vi "UDP_choosen_string_to_DBL.vi"(4 "main ID":i32, 5 "secondary ID":i32, 6 "Data to read":T1, 7 "input string":string) -> (3 "output number":dbl)   [LabVIEW 2012]
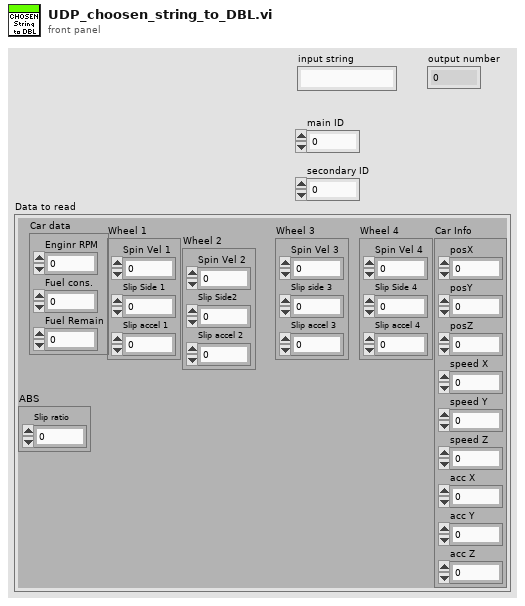
[diagram p1: front panel]
types:
  T1 = cluster{"Car data ":cluster{"Enginr RPM":dbl, "Fuel cons.":dbl, "Fuel Remain":dbl}, "Wheel 1":cluster{"Spin Vel 1":dbl, "Slip Side 1":dbl, "Slip accel 1":dbl}, "Wheel 2":cluster{"Spin Vel 2":dbl, "Slip Side2":dbl, "Slip accel 2":dbl}, "Wheel 3":cluster{"Spin Vel 3":dbl, "Slip side 3":dbl, "Slip accel 3":dbl}, "Wheel 4":cluster{"Spin Vel 4":dbl, "Slip Side 4":dbl, "Slip accel 4":dbl}, "Car Info":cluster{"posX":dbl, "posY":dbl, "posZ":dbl, "speed X":dbl, "speed Y":dbl, "speed Z":dbl, "acc X":dbl, "acc Y":dbl, "acc Z":dbl}, "ABS":cluster{"Slip ratio":dbl}}
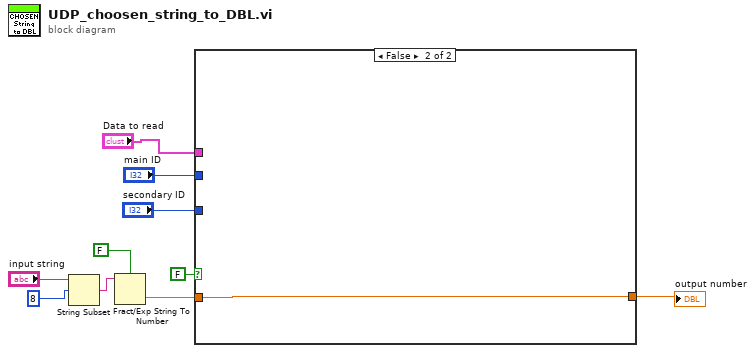
[diagram p0: block diagram]
diagram:
  n1 = String Subset(string="input string", offset (0)=8 ("offset")) -> (substring=w9:string)  [unwired: 1 in]
  n2 = Fract/Exp String To Number(use system decimal point (T)=FALSE, string=w9) -> (number=w6:dbl)  [unwired: 2 in, 1 out]
  n3 = case shown="False" FALSE {
    tunnel: w6 -> [w11 w12]
    tunnel: [w11 w12] -> w7
    tunnel: "main ID" -> [_ _]
    tunnel: "secondary ID" -> [_ _]
    tunnel: "Data to read" -> [_ _]
    frame True {
    }
    frame False {
    }
  }
  "output number" <- w7
